vi "categorize.vi"(10 "候補配列（正規表現）":string[](array[string]), 11 "入力文字列":string) -> (3 "結果":string)   [LabVIEW 2017]
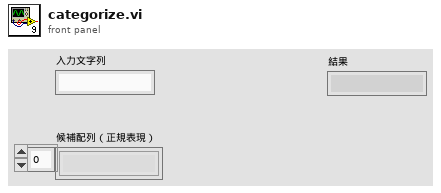
[diagram p1: front panel]
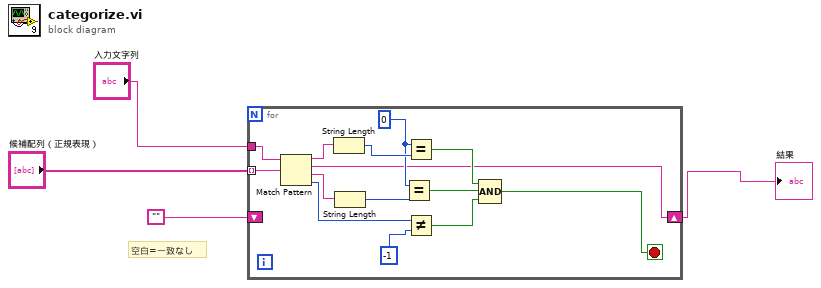
[diagram p0: block diagram]
diagram:
  # "空白=一致なし"
  n1 = for {
    tunnel: "候補配列（正規表現）" -> [w18] mode=indexing
    tunnel: "入力文字列" -> [w17]
    shift-right: [w5] -> w1
    shift-left: "" -> [_]
    stop <- w6 stop-if-true
    w13 = 0
    n2 = Match Pattern(string=w17, regular expression=w18) -> (before substring=w16:string, match substring=w5:string, after substring=w15:string, offset past match=w10:i32)  [unwired: 1 in]
    n3 = String Length(string=w16) -> (length=w14:i32)
    n4 = String Length(string=w15) -> (length=w12:i32)
    n5 = Equal?(x=w13, y=w12) -> (x = y?=w8:bool)
    n6 = Equal?(x=w13, y=w14) -> (x = y?=w9:bool)
    n7 = Not Equal?(x=w10, y=-1) -> (x != y?=w7:bool)
    n8 = Compound Arithmetic op=AND ("複合演算")(w9, w8, w7) -> (w6:bool)
  }
  "結果" <- w1
